vi "TA_Read_Data_2.vi"(0 "File Path":path=path "\\\\Mac\\Home/Desktop/fs-TA/Data/demo_fsta.dat") -> (1 "raw data":dbl[][](array[numeric]) format="%#_8g", 3 "size(delay time)":i32, 4 "size (wavelength)":i32, 5 "delay time (ps)":dbl[](array[numeric]), 6 "wavelength (nm)":dbl[](array[numeric]), 7 "deltaA (mOD)":dbl[][](array[numeric]))   [LabVIEW 2025]
uses:
  <vilib>/Utility/file.llb/Read Delimited Spreadsheet (DBL).vi
panel:
  out "size (deltaA)":i32[](array[numeric])
  out "size (raw data)":i32[](array[numeric])
  in  "delimiter (\\t tab; , comma)":string="\t"
  in  "transpose? (F)":bool
  in  "max characters/row  (no limit:0)":i32
  in  "start of read offset (chars.:0)":i32
  in  "number of rows (all:-1)":i32=-1
  in  "format (%.8f)":string="%.8f"
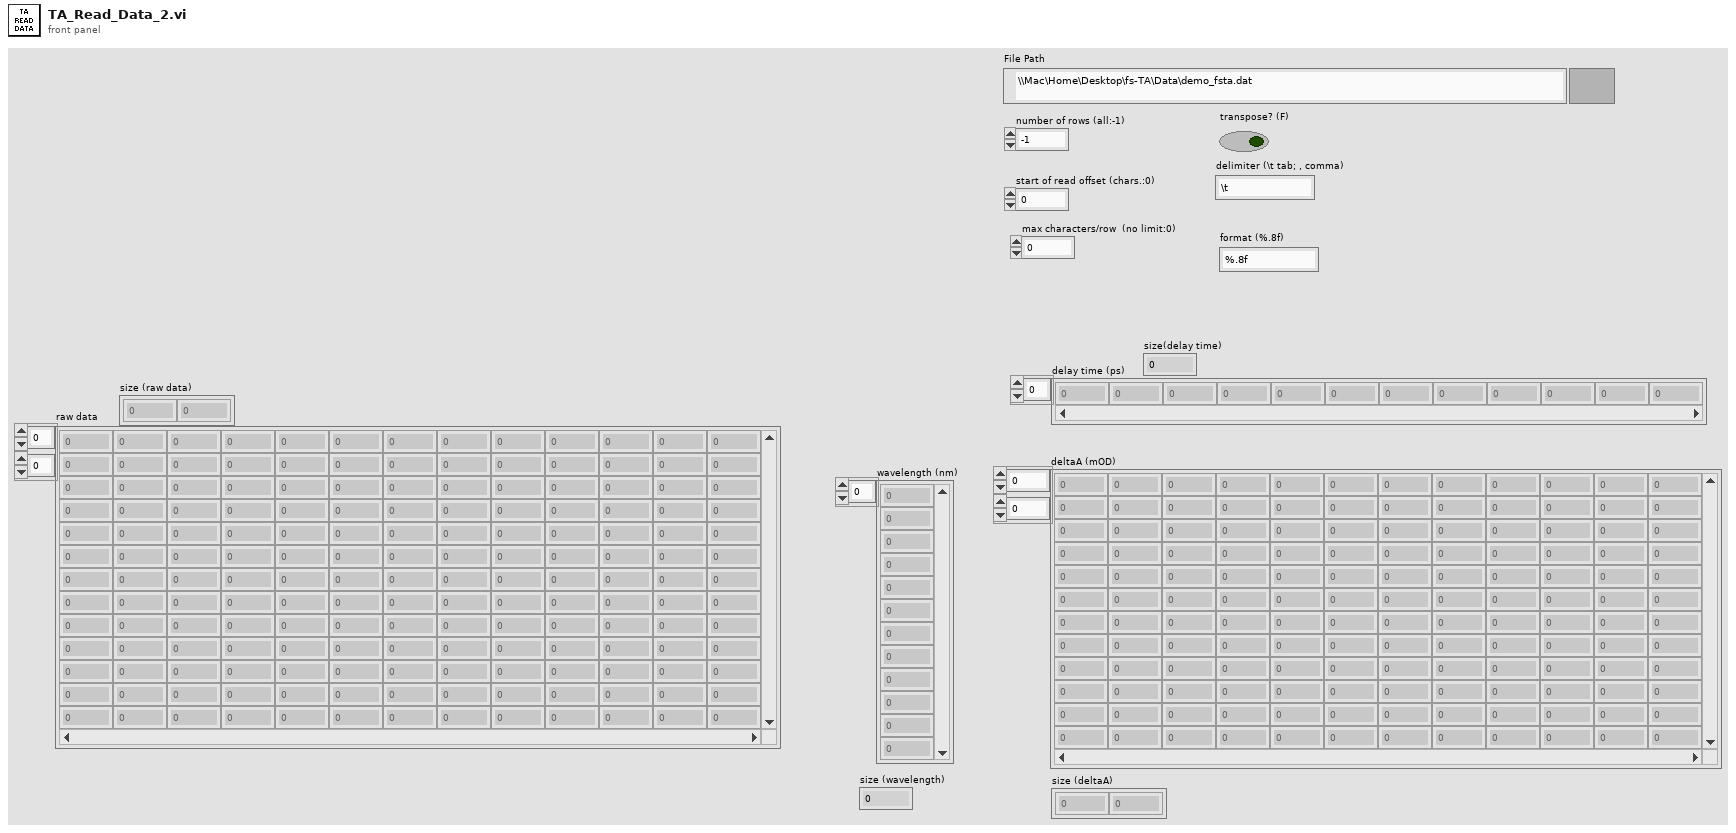
[diagram p1: front panel]
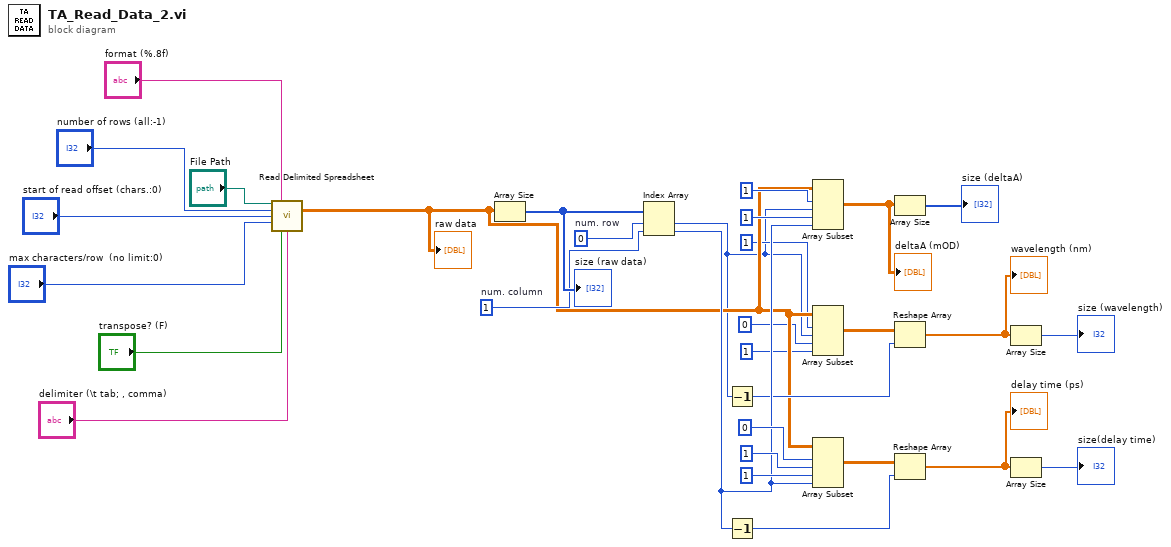
[diagram p0: block diagram]
diagram:
  w16 = 1  # num. column
  w24 = 0  # num. row
  n1 = call-poly <vilib>:"Read Delimited Spreadsheet.vi"("file path (dialog if empty)"="File Path", "format (%.3f)"="format (%.8f)", "number of rows (all:-1)"="number of rows (all:-1)", "start of read offset (chars.:0)"="start of read offset (chars.:0)", "max characters/row  (no limit:0)"="max characters/row  (no limit:0)", "transpose? (F)"="transpose? (F)", "delimiter (\\t)"="delimiter (\\t tab; , comma)") -> ("all rows"=w8:dbl[][])  [unwired: 3 in, 5 out]
  "raw data" <- w8
  n2 = Array Size(array=w8) -> (size(s)=w20:i32[])
  "size (raw data)" <- w20
  n3 = Index Array "Index Array"(array=w20, index #1=w24, index #2=w16) -> (element #1=w4:i32, element #2=w13:i32)
  n4 = Decrement(x=w4) -> (x-1=w11:i32)
  n5 = Decrement(x=w13) -> (x-1=w12:i32)
  n6 = Array Subset "Array Subset"(array=w8, index (row)=1 ("index"), length (row)=w4, index (col)=1 ("index"), length (col)=w13) -> (w1:dbl[][])
  "deltaA (mOD)" <- w1
  n7 = Array Subset "Array Subset"(array=w8, index (row)=1 ("index"), length (row)=w4, index (col)=0 ("index"), length (col)=1 ("length")) -> (w9:dbl[][])
  n8 = Array Subset "Array Subset"(array=w8, index (row)=0 ("index"), length (row)=1 ("length"), index (col)=1 ("index"), length (col)=w13) -> (w19:dbl[][])
  n9 = Array Size(array=w1) -> (size(s)=→"size (deltaA)":i32[])
  n10 = Reshape Array "Reshape Array"(w9, w11) -> (w2:dbl[])
  "wavelength (nm)" <- w2
  n11 = Reshape Array "Reshape Array"(w19, w12) -> (w3:dbl[])
  "delay time (ps)" <- w3
  n12 = Array Size(array=w2) -> (size(s)=→"size (wavelength)":i32)
  n13 = Array Size(array=w3) -> (size(s)=→"size(delay time)":i32)
